vi "Save Data.vi"(3 "Data Buffer":sgl[](array[numeric]) format="%.2f", 4 "Config Cluster":T2={"Pressure Setpoint"=20.0, "Deadband"=2.0, "Data Read Rate"=10.0, "Data Location"=1, "# Points to Ave."=2, "Data Storage"=FALSE, "Data Storage Rate"=10.0, "Data Path"=path "", "TR #"="", "Comp. ID"="", "Reset Buffer"=FALSE, "Reponse Time"=2.0} {"Reponse Time" min=0.0 max=10.0 format="%.1f"; "Data Storage Rate" min=1.0 max=100000.0 format="%<%H:%M:%S%0u>t"; "# Points to Ave." min=1 max=10000; "Data Location" min=1 max=10; "Data Read Rate" min=0.1 max=3600.0 format="%.1f"; "Deadband" format="%.2f"; "Pressure Setpoint" format="%.2f"}, 5 "Pr. Cal.":T1={"Model"="", "Gage #"="", "Cal Date"="", "Eng. Units"=[0.0, 0.0, 0.0, 0.0, 0.0, 0.0], "Amps"=[0.0, 0.0, 0.0, 0.0, 0.0, 0.0], "# Cal Points"=5, "Offset"=0.0, "Slope"=0.0, "Units"="psi", "Master Gage #"=""} {"Slope" format="%.4f"; "Offset" format="%.4f"; "# Cal Points" min=2 max=6; "Amps" format="%.3f"; "Eng. Units" format="%.3f"}) -> ()   [LabVIEW 2013]
panel:
  # "(2-6)"
  # "(0.1-3600)"
  # "(0-10)"
  # "(1-10000)"
  # "(1-10)"
  # "(hh:mm:ss)"
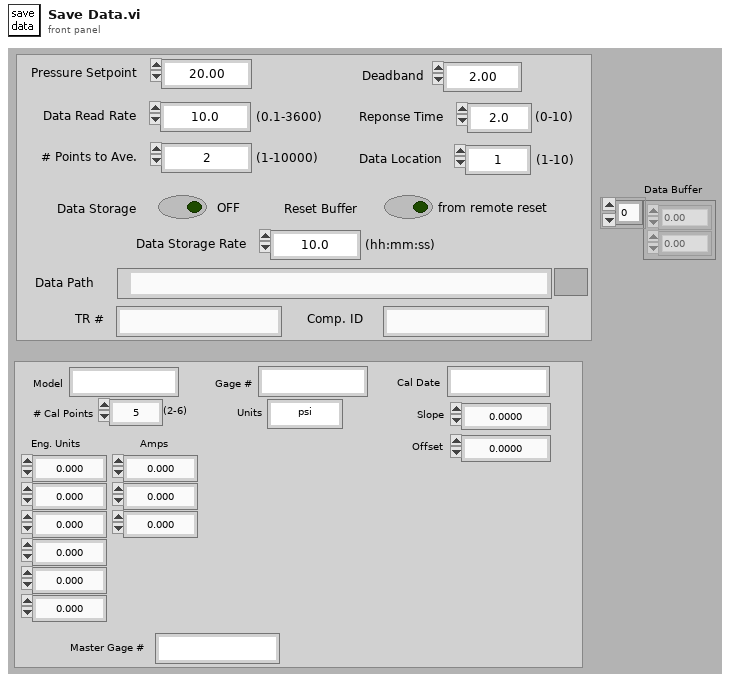
[diagram p1: front panel]
types:
  T1 = cluster{"Model":string, "Gage #":string, "Cal Date":string, "Eng. Units":sgl[], "Amps":sgl[], "# Cal Points":u32, "Offset":sgl, "Slope":sgl, "Units":string, "Master Gage #":string}
  T2 = cluster{"Pressure Setpoint":dbl, "Deadband":dbl, "Data Read Rate":dbl, "Data Location":i32, "# Points to Ave.":i32, "Data Storage":bool, "Data Storage Rate":dbl, "Data Path":path, "TR #":string, "Comp. ID":string, "Reset Buffer":bool, "Reponse Time":dbl}
  T3 = enum16{"open", "replace", "create", "open or create", "replace or create", "replace or create with confirmation"}
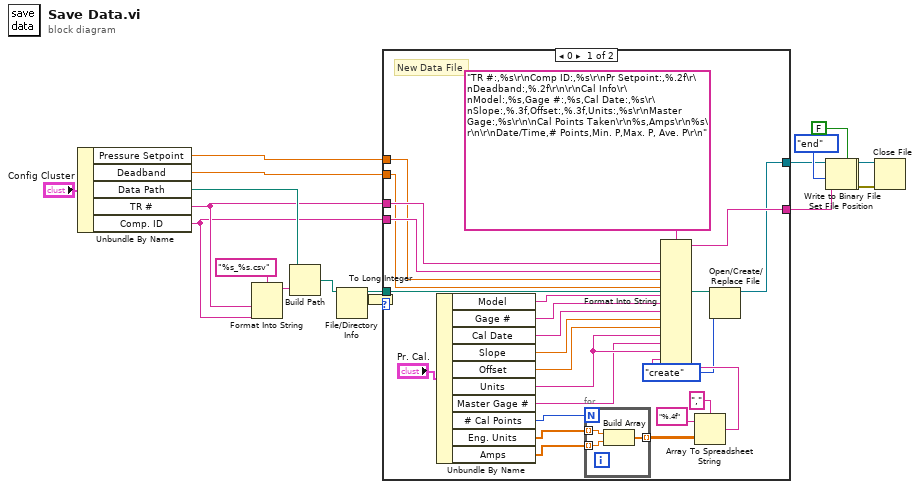
[diagram p0: block diagram]
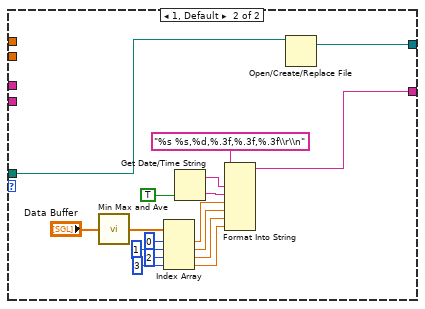
[diagram p2: hidden frame]
diagram:
  n1 = Unbundle By Name("Config Cluster") -> ("Pressure Setpoint"=w14:dbl, "Deadband"=w13:dbl, "Data Path"=w18:path, "TR #"=w12:string, "Comp. ID"=w11:string)
  n2 = Format Into String(format string="%s_%s.csv" ("Format String"), w12, w11) -> (resulting string=w19:string)  [unwired: 2 in, 1 out]
  n3 = Build Path(base path=w18, name or relative path=w19) -> (appended path=w16:path)
  n4 = File/Directory Info(path=w16) -> (path out=w7:path, size=w4:i64)  [unwired: 1 in, 5 out]
  n5 = To Long Integer(number=w4) -> (32bit integer=w15:i32)
  n6 = case shown="0" w15 {
    tunnel: w14 -> [w41 _]
    tunnel: w13 -> [w40 _]
    tunnel: w12 -> [w43 _]
    tunnel: w11 -> [w42 _]
    tunnel: [w39 w48] -> w5
    tunnel: w7 -> [w38 w64]
    tunnel: [w37 w63] -> w6
    frame 0 {
      # "New Data File"
      n7 = Unbundle By Name("Pr. Cal.") -> ("Model"=w35:string, "Gage #"=w34:string, "Cal Date"=w33:string, "Slope"=w32:sgl, "Offset"=w31:sgl, "Units"=w23:string, "Master Gage #"=w22:string, "# Cal Points"=w27:u32, "Eng. Units"=w26:sgl[], "Amps"=w25:sgl[])
      n8 = for {
        N: w27 -> [_]
        tunnel: w26 -> [w47] mode=indexing
        tunnel: w25 -> [w46] mode=indexing
        tunnel: [w45] -> w30 mode=indexing
        n9 = Build Array(w47, w46) -> (w45:sgl[])
      }
      n10 = Array To Spreadsheet String(delimiter (Tab)=",", array=w30, 3:"%.4f" ("format string")) -> (spreadsheet string=w24:string)
      n11 = Format Into String(format string="TR #:,%s\r\nComp ID:,%s\r\nPr Setpoint:,%.2f\r\nDeadband:,%.2f\r\n\r\nCal Info\r\nModel:,%s,Gage #:,%s,Cal Date:,%s\r\nSlope:,%.3f,Offset:,%.3f,Units:,%s\r\nMaster Gage:,%s\r\n\nCal Points Taken\r\n%s,Amps\r\n%s\r\n\r\nDate/Time,# Points,Min. P,Max. P, Ave. P\r\n", w43, w42, w41, w40, w35, w34, w33, w32, w31, w23, w22, w23, w24) -> (resulting string=w39:string)  [unwired: 2 in, 1 out]
      n12 = Open/Create/Replace File(file path (use dialog)=w38, operation (0:open)=T3."create") -> (refnum out=w37:refnum<file>)  [unwired: 4 in, 2 out]
    }
    frame 1, Default {
      n13 = call "Min Max and Ave.vi"("Data In"="Data Buffer") -> ("# Pts, Min, Max, Ave."=w57:sgl[])  [unwired: 1 in, 1 out]
      n14 = Index Array(array=w57, index #1=0 ("Index"), index #2=1 ("Index"), index #3=2 ("Index"), index #4=3 ("Index")) -> (element #1=w59:sgl, element #2=w58:sgl, element #3=w55:sgl, element #4=w61:sgl)
      n15 = Get Date/Time String(want seconds? (F)=TRUE) -> (date string=w50:string, time string=w49:string)  [unwired: 2 in]
      n16 = Format Into String(format string="%s %s,%d,%.3f,%.3f,%.3f\\r\\n" ("Format String"), w50, w49, w59, w58, w55, w61) -> (resulting string=w48:string)  [unwired: 2 in, 1 out]
      n17 = Open/Create/Replace File(file path (use dialog)=w64) -> (refnum out=w63:refnum<file>)  [unwired: 5 in, 2 out]
    }
  }
  n18 = Set File Position(refnum=w6, from (0:start)=enum16{"start", "end", "current"}."end" ("pos mode (0:2)")) -> (refnum out=w3:refnum<file>, error out=w2:errorcluster)  [unwired: 2 in]
  n19 = Write to Binary File(file (use dialog)=w3, data=w5, error in=w2, 5:FALSE ("prepend array or string size? (T)")) -> (refnum out=w8:refnum<file>, error out=w9:errorcluster)  [unwired: 2 in, 1 out]
  n20 = Close File(refnum=w8, error in=w9) -> ()  [unwired: 2 out]
